vi "ex7-10.vi"() -> ()   [LabVIEW 2013]
panel:
  out "output array":dbl[](array[numeric])
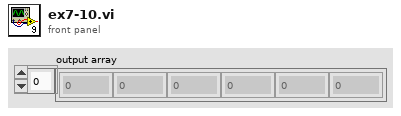
[diagram p1: front panel]
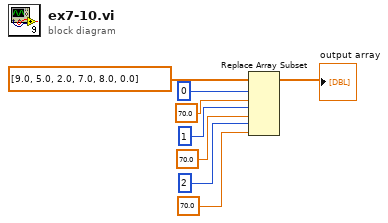
[diagram p0: block diagram]
diagram:
  n1 = Replace Array Subset(array=dbl[] [9.0, 5.0, 2.0, 7.0, 8.0, 0.0], new element #1=70.0 ("new element/subarray"), index #1=0 ("index"), new element #2=70.0 ("new element/subarray"), index #2=1 ("index"), new element #3=70.0 ("new element/subarray"), index #3=2 ("index")) -> (→"output array":dbl[])
